vi "F Dwf Device Open.vi"(8 "error in (no error)":errorcluster, 10 "phdwf":i32, 11 "idxDevice":i32) -> (0 "error out":errorcluster, 2 "phdwf out":i32, 3 "function return":i32)   [LabVIEW 2024, in "Olasdwf.lvlib"]
doc: "DWFAPI int FDwfDeviceOpen(int idxDevice, HDWF *phdwf);"
uses:
  Olasdwf.lvlib
  Windows/System32/dwf.dll
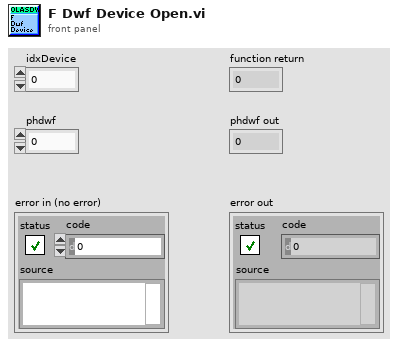
[diagram p1: front panel]
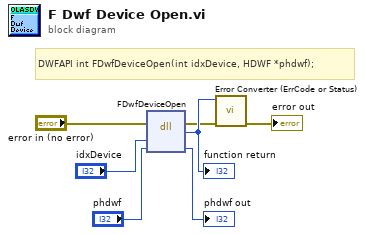
[diagram p0: block diagram]
diagram:
  # "DWFAPI int FDwfDeviceOpen(int idxDevice, HDWF *phdwf);"
  n1 = dll-call lib="/Windows/System32/dwf.*" fn="FDwfDeviceOpen"(error in="error in (no error)", "idxDevice"="idxDevice", "phdwf"="phdwf") -> (error out=w2:errorcluster, w7:i32, "phdwf"=→"phdwf out":i32)  [unwired: 3 in, 1 out]
  "function return" <- w7
  n2 = call "Error Converter (ErrCode or Status).vi"("error in (no error)"=w2, "error code"=w7) -> ("error out"=→"error out":errorcluster)  [unwired: 9 in]
